vi "Read Exe WriteDate.vi"(1 "File Path in":path) -> (0 "Last Write Time":string)   [LabVIEW 2020]
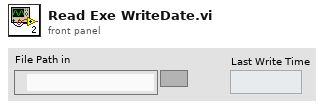
[diagram p1: front panel]
types:
  T1 = cluster{"Year":u16, "Month":u16, "DayOfWeek":u16, "Day":u16, "Hour":u16, "Minute":u16, "Seconds":u16, "Milliseconds":u16}
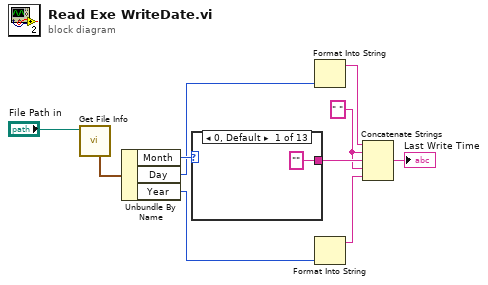
[diagram p0: block diagram]
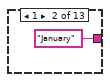
[diagram p2: hidden frame]
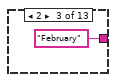
[diagram p3: hidden frame]
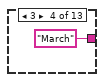
[diagram p4: hidden frame]
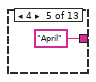
[diagram p5: hidden frame]
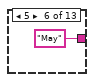
[diagram p6: hidden frame]
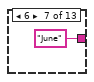
[diagram p7: hidden frame]
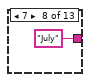
[diagram p8: hidden frame]
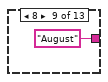
[diagram p9: hidden frame]
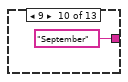
[diagram p10: hidden frame]
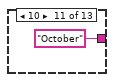
[diagram p11: hidden frame]
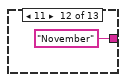
[diagram p12: hidden frame]
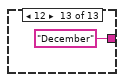
[diagram p13: hidden frame]
diagram:
  w4 = " " ("string")
  n1 = call "Get File Info.vi"("File Path in"="File Path in") -> ("Last Write Time"=w9:T1)  [unwired: 4 in, 6 out]
  n2 = Unbundle By Name(w9) -> ("Month"=w8:u16, "Day"=w7:u16, "Year"=w3:u16)
  n3 = case shown="0, Default" w8 {
    tunnel: ["" "January" "February" "March" "April" "May" "June" "July" "August" "September" "October" "November" "December"] -> w5
    frame 0, Default {
    }
    frame 1 {
    }
    frame 2 {
    }
    frame 3 {
    }
    frame 4 {
    }
    frame 5 {
    }
    frame 6 {
    }
    frame 7 {
    }
    frame 8 {
    }
    frame 9 {
    }
    frame 10 {
    }
    frame 11 {
    }
    frame 12 {
    }
  }
  n4 = Format Into String(w7) -> (resulting string=w6:string)  [unwired: 3 in, 1 out]
  n5 = Format Into String(w3) -> (resulting string=w2:string)  [unwired: 3 in, 1 out]
  n6 = Concatenate Strings(w6, w4, w5, w4, w2) -> (→"Last Write Time":string)
